vi "Simulator_0720.vi"() -> ()   [LabVIEW 2017]
doc: "This example demonstrates how to continuously acquire buffered voltage measurements using a DAQmx device.\n\nFor instructions on how to connect your signals to the DAQ device, refer to your device documentation."
uses:
  <vilib>/Utility/error.llb/DialogType.ctl
  <vilib>/DAQmx/read.llb/DAQmx Read (Analog 1D Wfm NChan NSamp).vi
  <vilib>/Analysis/5stat.llb/RMS (DBL).vi
  <vilib>/Analysis/polynomials.llb/Polynomial Roots (DBL).vi
  <vilib>/DAQmx/miscellaneous.llb/DAQmx Fill In Error Info.vi
  <vilib>/express/express shared/transition.llb/Dynamic To Waveform Array.vi
  <vilib>/express/express arith-compare/Formula/Block/exnFormulaBlock how many pts in the wave.vi
  <vilib>/express/express shared/ex_Modify Signal Name.vi
  <vilib>/express/express shared/transition.llb/Waveform Array To Dynamic.vi
  <vilib>/measure/maspectr.llb/FFT Power Spectrum and PSD for N Chan.vi
  <vilib>/measure/mascope.llb/Cycle Average and RMS N chan.vi
  <vilib>/express/express arith-compare/Formula/XNode/ExpressFormulaBlockNode.xnode
  <vilib>/measure/NI_MAPro.lvlib
  SetupDAQ.vi
  <vilib>/Analysis/NI_AALPro.lvlib
  <vilib>/gmath/NI_Gmath.lvlib
panel:
  out "Roots":cdb[](array[numeric]) caption="근"
  in  "P(x)":dbl[](array[numeric])
  out "A,B,C,D Filtering Signal 9":dynamicdata(graph) caption="A,B Filtering Signal"
  out "A,B,C,D Filtering Signal 8":dbl(graph) caption="A,B Filtering Signal"
  out "슬라이드 3":dbl(slide) scale=1.5..0.5
  out "A,B,C,D Filtering Signal 7":dynamicdata(graph) caption="A,B Filtering Signal"
  out "Raw Signal 4":dynamicdata(graph)
  out "Raw Signal 3":waveform(dbl)[](graph)
  out "A,B,C,D Filtering Signal 3":dynamicdata(graph) caption="A,B Filtering Signal"
  out "A,B,C,D Filtering Signal 2":dynamicdata(graph) caption="A,B Filtering Signal"
  out "슬라이드 2":dbl(slide) scale=-0.6..3.0
  out "슬라이드":dbl(slide) scale=1.0..3.5
  out "2.5HZ-Step":dynamicdata(graph)
  in  "동작 라벨":T1(radio)
  in  "Sensor C Channel 2":tag="Dev2/ai0"
  in  "Sensor D Channel 2":tag="Dev2/ai1"
  in  "Terminal config 2":i32(ring)=10083 items=["default"=-1, "RSE"=10083, "NRSE"=10078, "Differential"=10106, "Pseudodifferential"=12529]
  out "55-65(A)":dynamicdata(graph)
  out "10-20(A)":dynamicdata(graph)
  out "A,B,C,D Filtering Signal":dynamicdata(graph) caption="A,B Filtering Signal"
  out "Differential Signal A-B, C-D":dynamicdata(graph)
  in  "number of averages":u32=1
  out "Power Spectrum / PSD":cluster{"f0":dbl, "df":dbl, "magnitude":dbl[]}[](graph)
  out "detected amplitudes 2":dbl(graph)=1.1331379876254155
  out "detected frequencies 2":dbl(graph)
  out "detected frequencies":dbl[](array[numeric])=[60.0, 60.0]
  out "detected amplitudes":dbl[](array[numeric])=[1.1331379876254155, 0.40633237156802526]
  out "Raw Signal 2":waveform(dbl)[](graph)
  out "Raw Signal":waveform(dbl)[](graph)
  in  "Sensor B Channel":tag="Dev2/ai1"
  in  "Sensor A Channel":tag="Dev2/ai0"
  in  "Terminal config":i32(ring)=10083 items=["default"=-1, "RSE"=10083, "NRSE"=10078, "Differential"=10106, "Pseudodifferential"=12529]
  in  "rate":dbl=5000.0
  out "FFT Power Spectrum":cluster{"f0":dbl, "df":dbl, "magnitude":dbl[]}[](graph)
  in  "Stop":bool
  in  "Number of Samples":i32=100
  # "Channel Settings"
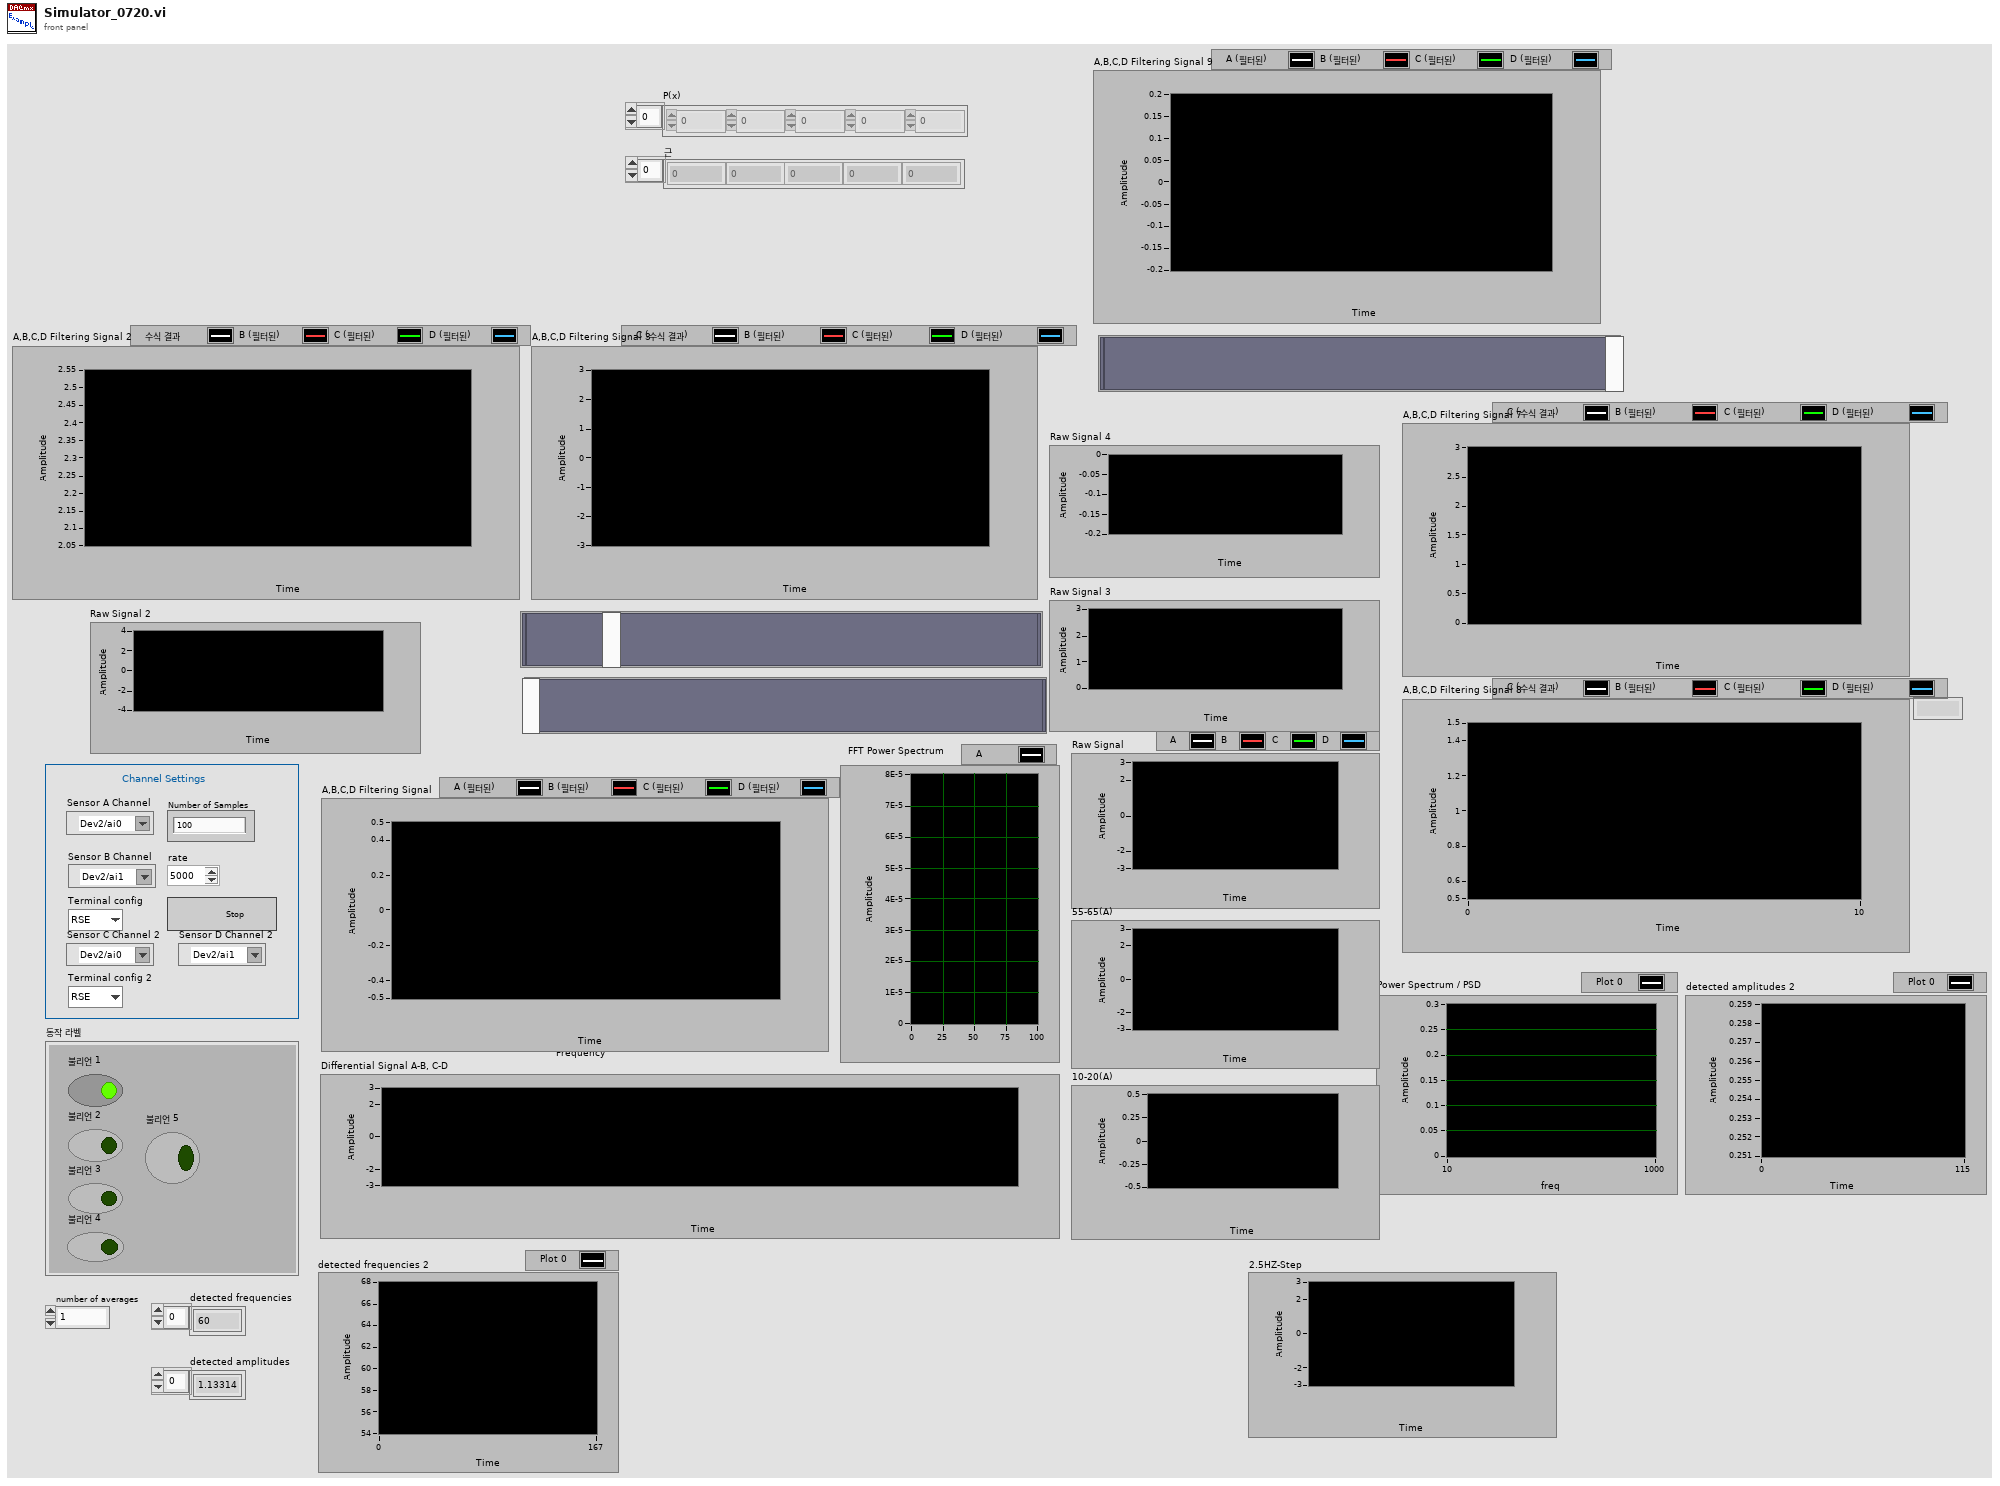
[diagram p1: front panel]
types:
  T1 = enum32{"불리언 1", "불리언 2", "불리언 3", "불리언 4", "불리언 5"}
  T2 = typedef "DialogType.ctl" = u16
  T3 = cluster{"averaging mode":enum16{"No averaging", "Vector averaging", "RMS averaging", "Peak hold"}, "weighting mode":enum16{"Linear", "Exponential"}, "number of averages":u32}
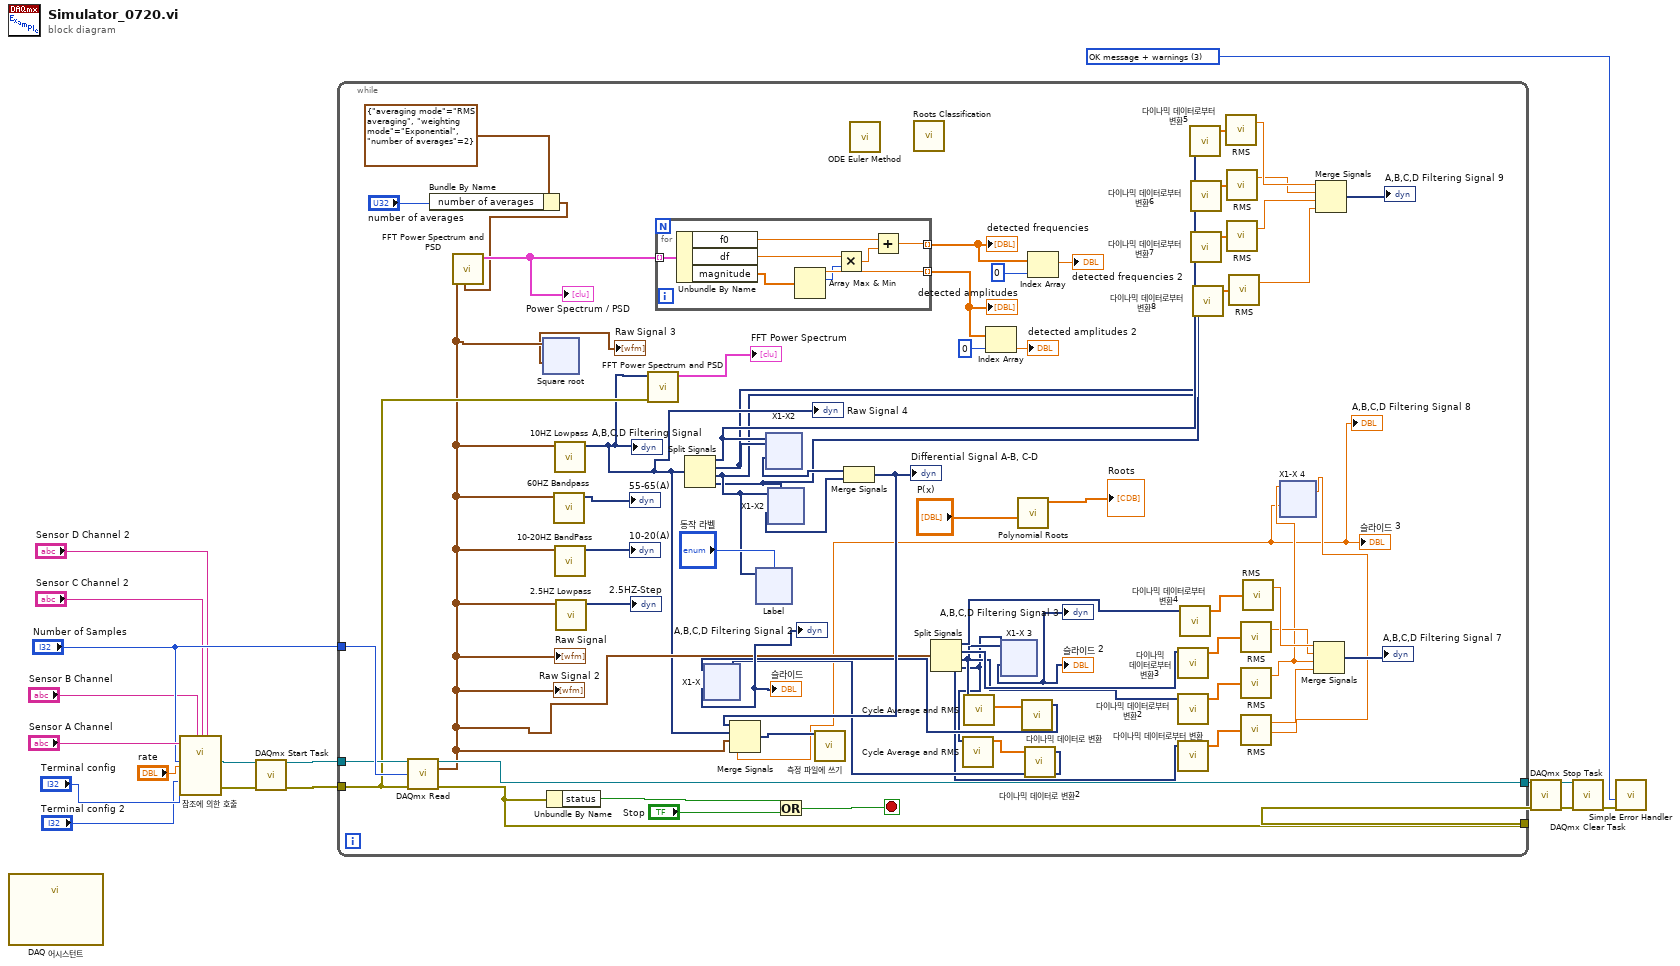
[diagram p0: block diagram]
diagram:
  w11 = T2 3 items=["no dialog", "OK message", "continue or stop message", "OK message + warnings", "continue/stop + warnings"] ("type of dialog (OK msg:1)")
  n1 = call "DAQ 어시스턴트"() -> ()  [unwired: 12 in]
  n2 = call-by-ref "참조에 의한 호출"("number of samples"="Number of Samples", "rate"="rate", "input terminal configuration"="Terminal config", "input terminal configuration 2"="Terminal config 2", "physical channel"="Sensor A Channel", "physical channel 2"="Sensor B Channel", "physical channel 3"="Sensor C Channel 2", "physical channel 4"="Sensor D Channel 2") -> ("task out"=w7:refnum<k21>, "error out"=w6:errorcluster)  [unwired: 12 in, 2 out]
  n3 = call <vilib>:"DAQmx Start Task.vi"("task/channels in"=w7, "error in"=w6) -> ("task out"=w18:refnum<k21>, "error out"=w17:errorcluster)  [unwired: 12 in]
  n4 = while "While 루프" {
    tunnel: w18 -> [w78]
    tunnel: w17 -> [w77]
    tunnel: [w83] -> w15
    tunnel: [w81] -> w14
    tunnel: "Number of Samples" -> [w79]
    stop <- w80 stop-if-true
    n5 = call-poly <vilib>:"DAQmx Read.vi"("task/channels in"=w78, "number of samples per channel"=w79, "error in"=w77) -> ("task out"=w83:refnum<k21>, "data"=w49:waveform(dbl)[], "error out"=w81:errorcluster)  [unwired: 10 in]
    "Raw Signal" <- w49
    "Raw Signal 2" <- w49
    n6 = Bundle By Name ("이름으로 묶기")(cluster=T3 {"averaging mode"=enum."RMS averaging", "weighting mode"=enum."Exponential", "number of averages"=2} ("averaging parameters"), "number of averages"="number of averages") -> (w57:T3)
    n7 = call-poly <vilib>:"FFT Power Spectrum and PSD.vi"("averaging parameters"=w57, "time signals"=w49) -> ("Power Spectrum / PSD"=w59:cluster{"f0":dbl, "df":dbl, "magnitude":dbl[]}[])  [unwired: 6 in, 3 out]
    "Power Spectrum / PSD" <- w59
    n8 = xnode "Square root"("X1"=w49) -> ("결과"=→"Raw Signal 3":waveform(dbl)[])  [unwired: 1 in, 1 out]
    n9 = Unbundle By Name(w81) -> ("status"=w68:bool)
    n10 = call "60HZ Bandpass"("Signal"=w49) -> ("Filtered Signal"=→"55-65(A)":dynamicdata)  [unwired: 9 in, 1 out]
    n11 = call "10HZ Lowpass"("Signal"=w49) -> ("Filtered Signal"=w47:dynamicdata)  [unwired: 9 in, 1 out]
    "A,B,C,D Filtering Signal" <- w47
    "Raw Signal 4" <- w47
    n12 = call "10-20HZ BandPass"("Signal"=w49) -> ("Filtered Signal"=→"10-20(A)":dynamicdata)  [unwired: 9 in, 1 out]
    n13 = call "2.5HZ Lowpass"("Signal"=w49) -> ("Filtered Signal"=→"2.5HZ-Step":dynamicdata)  [unwired: 9 in, 1 out]
    n14 = call-poly <vilib>:"FFT Power Spectrum and PSD.vi"("error in (no error)"=w77, "time signals"=w47) -> ("Power Spectrum / PSD"=→"FFT Power Spectrum":cluster{"f0":dbl, "df":dbl, "magnitude":dbl[]}[])  [unwired: 6 in, 3 out]
    n15 = for {
      tunnel: w59 -> [w922] mode=indexing
      tunnel: [w925] -> w74 mode=indexing
      tunnel: [w923] -> w71 mode=indexing
      n16 = Unbundle By Name(w922) -> ("f0"=w918:dbl, "df"=w924:dbl, "magnitude"=w921:dbl[])
      n17 = Array Max & Min(array=w921) -> (max value=w925:dbl, max index (indices)=w920:i32)  [unwired: 2 out]
      n18 = Multiply(x=w924, y=w920) -> (x*y=w919:dbl)
      n19 = Add(x=w918, y=w919) -> (x+y=w923:dbl)
    }
    "detected amplitudes" <- w74
    "detected frequencies" <- w71
    n20 = Split Signals(w47) -> (w39:dynamicdata, w37:dynamicdata, w35:dynamicdata, w33:dynamicdata)  [unwired: 4 in]
    n21 = xnode "Label"("X1"=w35, "X2"="동작 라벨") -> ()  [unwired: 1 in, 2 out]
    n22 = xnode "X1-X2"("X1"=w39, "X2"=w37) -> ("결과"=w64:dynamicdata)  [unwired: 1 in, 1 out]
    n23 = xnode "X1-X2"("X1"=w35, "X2"=w33) -> ("결과"=w63:dynamicdata)  [unwired: 1 in, 1 out]
    n24 = Or(x=w68, y="Stop") -> (x .or. y?=w80:bool)
    n25 = Merge Signals(w64, w63) -> (w61:dynamicdata)
    "Differential Signal A-B, C-D" <- w61
    n26 = call <vilib>:"ODE Euler Method.vi"() -> ()  [unwired: 7 in, 4 out]
    n27 = call <vilib>:"Roots Classification.vi"() -> ()  [unwired: 8 in, 4 out]
    n28 = Split Signals(w49) -> (w43:dynamicdata, w42:dynamicdata, w41:dynamicdata, w40:dynamicdata)  [unwired: 4 in]
    n29 = call-poly <vilib>:"Cycle Average and RMS.vi"("signal(s) in"=w40) -> ("cycle average"=w52:dbl[])  [unwired: 7 in, 3 out]
    n30 = call-poly <vilib>:"Cycle Average and RMS.vi"("signal(s) in"=w41) -> ("cycle RMS"=w51:dbl[])  [unwired: 7 in, 3 out]
    n31 = Index Array(array=w74, index=0) -> (element=→"detected amplitudes 2":dbl)
    n32 = xnode "X1-X 3"("X1"=w41, "X2"=w40) -> ("결과"=→"슬라이드 2" →"A,B,C,D Filtering Signal 3":dynamicdata)  [unwired: 1 in, 1 out]
    n33 = call-poly <vilib>:"Polynomial Roots.vi"("P(x)"="P(x)") -> ("Roots"=→"Roots":cdb[])  [unwired: 9 in, 1 out]
    n34 = call "다이나믹 데이터로 변환"("Array"=w51) -> ("Dynamic Data Type"=w54:dynamicdata)  [unwired: 3 in]
    n35 = call "다이나믹 데이터로 변환2"("Array"=w52) -> ("Dynamic Data Type"=w53:dynamicdata)  [unwired: 3 in]
    n36 = xnode "X1-X"("X1"=w54, "X2"=w53) -> ("결과"=→"슬라이드" →"A,B,C,D Filtering Signal 2":dynamicdata)  [unwired: 1 in, 1 out]
    n37 = Index Array(array=w71, index=0) -> (element=→"detected frequencies 2":dbl)
    n38 = call "다이나믹 데이터로부터 변환3"("Dynamic Data Type"=w42) -> ("Array"=w45:dbl[])  [unwired: 3 in]
    n39 = call "다이나믹 데이터로부터 변환2"("Dynamic Data Type"=w41) -> ("Array"=w46:dbl[])  [unwired: 3 in]
    n40 = call "다이나믹 데이터로부터 변환"("Dynamic Data Type"=w40) -> ("Array"=w50:dbl[])  [unwired: 3 in]
    n41 = call "다이나믹 데이터로부터 변환4"("Dynamic Data Type"=w43) -> ("Array"=w44:dbl[])  [unwired: 3 in]
    n42 = call "다이나믹 데이터로부터 변환5"("Dynamic Data Type"=w39) -> ("Array"=w38:dbl[])  [unwired: 3 in]
    n43 = call "다이나믹 데이터로부터 변환6"("Dynamic Data Type"=w37) -> ("Array"=w36:dbl[])  [unwired: 3 in]
    n44 = call "다이나믹 데이터로부터 변환7"("Dynamic Data Type"=w35) -> ("Array"=w34:dbl[])  [unwired: 3 in]
    n45 = call "다이나믹 데이터로부터 변환8"("Dynamic Data Type"=w33) -> ("Array"=w32:dbl[])  [unwired: 3 in]
    n46 = call-poly <vilib>:"RMS.vi"("X"=w38) -> ("rms value"=w31:dbl)  [unwired: 1 out]
    n47 = call-poly <vilib>:"RMS.vi"("X"=w36) -> ("rms value"=w30:dbl)  [unwired: 1 out]
    n48 = call-poly <vilib>:"RMS.vi"("X"=w34) -> ("rms value"=w29:dbl)  [unwired: 1 out]
    n49 = call-poly <vilib>:"RMS.vi"("X"=w32) -> ("rms value"=w28:dbl)  [unwired: 1 out]
    n50 = call-poly <vilib>:"RMS.vi"("X"=w45) -> ("rms value"=w24:dbl)  [unwired: 1 out]
    n51 = call-poly <vilib>:"RMS.vi"("X"=w46) -> ("rms value"=w23:dbl)  [unwired: 1 out]
    n52 = call-poly <vilib>:"RMS.vi"("X"=w50) -> ("rms value"=w22:dbl)  [unwired: 1 out]
    n53 = call-poly <vilib>:"RMS.vi"("X"=w44) -> ("rms value"=w25:dbl)  [unwired: 1 out]
    n54 = xnode "X1-X 4"("X1"=w23, "X2"=w22) -> ("결과"=w19:dbl)  [unwired: 1 in, 1 out]
    "슬라이드 3" <- w19
    "A,B,C,D Filtering Signal 8" <- w19
    n55 = Merge Signals(w61, w47, w49, w19) -> (w60:dynamicdata)
    n56 = call "측정 파일에 쓰기"("Signals"=w60) -> ()  [unwired: 16 in, 3 out]
    n57 = Merge Signals(w25, w24, w23, w22) -> (→"A,B,C,D Filtering Signal 7":dynamicdata)
    n58 = Merge Signals(w31, w30, w29, w28) -> (→"A,B,C,D Filtering Signal 9":dynamicdata)
  }
  n59 = call <vilib>:"DAQmx Stop Task.vi"("task/channels in"=w15, "error in"=w14) -> ("task out"=w12:refnum<k21>, "error out"=w13:errorcluster)  [unwired: 12 in]
  n60 = call <vilib>:"DAQmx Clear Task.vi"("task in"=w12, "error in"=w13) -> ("error out"=w16:errorcluster)  [unwired: 13 in]
  n61 = call <vilib>:"Simple Error Handler.vi"("type of dialog (OK msg:1)"=w11, "error in (no error)"=w16) -> ()  [unwired: 3 in, 5 out]
